vi "Motion-Move-Y.vi"(4 "Y Drive Acc/Speed/Velocity":string="MA1: A 10: V 20: AD 10: D ", 8 "error in (no error)":errorcluster, 10 "Y Coordinates":string="880000", 11 "Motion-ControlAll in":refnum<class "Motion-ControlAll.lvclass">) -> (0 "error out":errorcluster, 3 "Motion-ControlAll out":refnum<class "Motion-ControlAll.lvclass">)   [LabVIEW 2013, in "Motion-ControlAll.lvclass"]
uses:
  Motion-ControlAll.lvclass
  Motion-ControlAll.lvclass/Motion-ControlAll.ctl
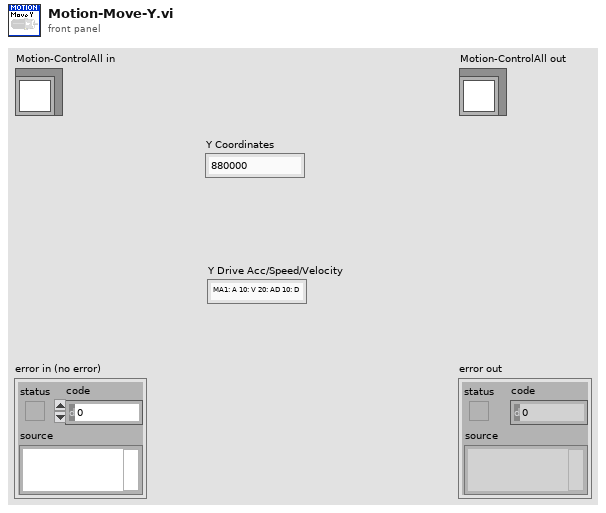
[diagram p1: front panel]
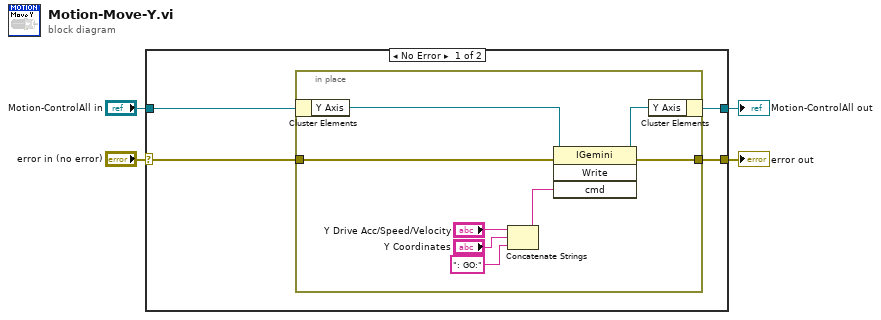
[diagram p0: block diagram]
diagram:
  n1 = case shown="No Error" "error in (no error)" {
    selector: "error in (no error)" -> [w7 w18]
    tunnel: [w5 w18] -> w3
    tunnel: [w6 w17] -> w1
    tunnel: "Motion-ControlAll in" -> [w8 w17]
    frame No Error {
      n2 = in-place {
        in-place-border: w7 -> [w12]
        in-place-border: [w9] -> w5
        n3 = in-place-cluster #1(w8) -> ("Y Axis"=w11:refnum<k7>)
        n4 = Concatenate Strings("Y Drive Acc/Speed/Velocity", "Y Coordinates", ": GO:" ("string")) -> (w16:string)
        n5 = invoke class="IGemini" method="Write"(reference=w11, error in=w12, "cmd"=w16) -> (reference out=w10:refnum<k7>, error out=w9:errorcluster)  [unwired: 1 in, 2 out]
        n6 = in-place-cluster #1("Y Axis"=w10) -> (w6:refnum<class "Motion-ControlAll.lvclass">)
      }
    }
    frame Error {
    }
  }
  "error out" <- w3
  "Motion-ControlAll out" <- w1
